vi "GetWhereIsMouseClick.vi"(10 "Coords":T1, 11 "XYGraph输入":refnum<vi>) -> (3 "WhereIsMouse":T2(ring))   [LabVIEW 2015]
uses:
  <vilib>/Utility/miscctls.llb/LVPoint32TypeDef.ctl
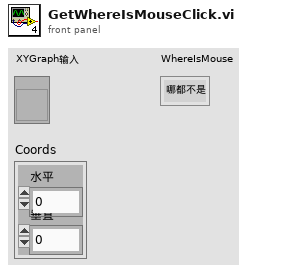
[diagram p1: front panel]
types:
  T1 = typedef "LVPoint32TypeDef.ctl" = cluster{"Horizontal":i32, "Vertical":i32}
  T2 = enum16{"哪都不是", "在曲线上", "在X轴上", "在单Y轴上", "在绘图区域但非曲线上", "在绘图区域上方", "在图例上"}
  T3 = enum16{"哪都不是", "在曲线上", "在X轴上", "在单Y轴上", "在绘图区域但非曲线上"}
  T4 = typedef "LVRectTypeDef.ctl" = cluster{"Left":i16, "Top":i16, "Right":i16, "Bottom":i16}
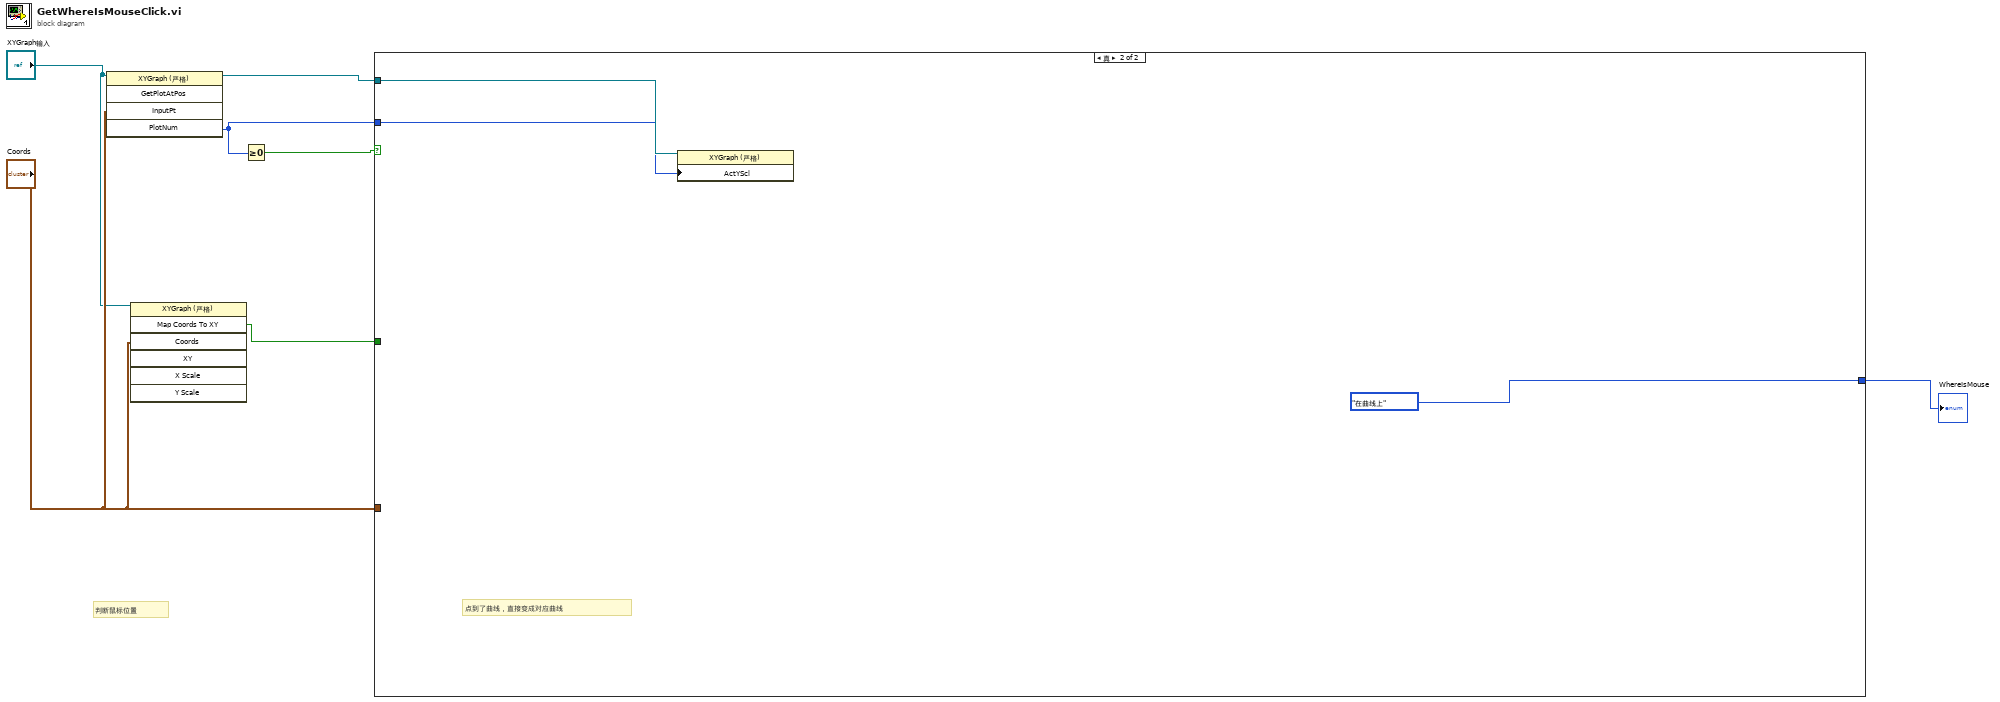
[diagram p0: block diagram]
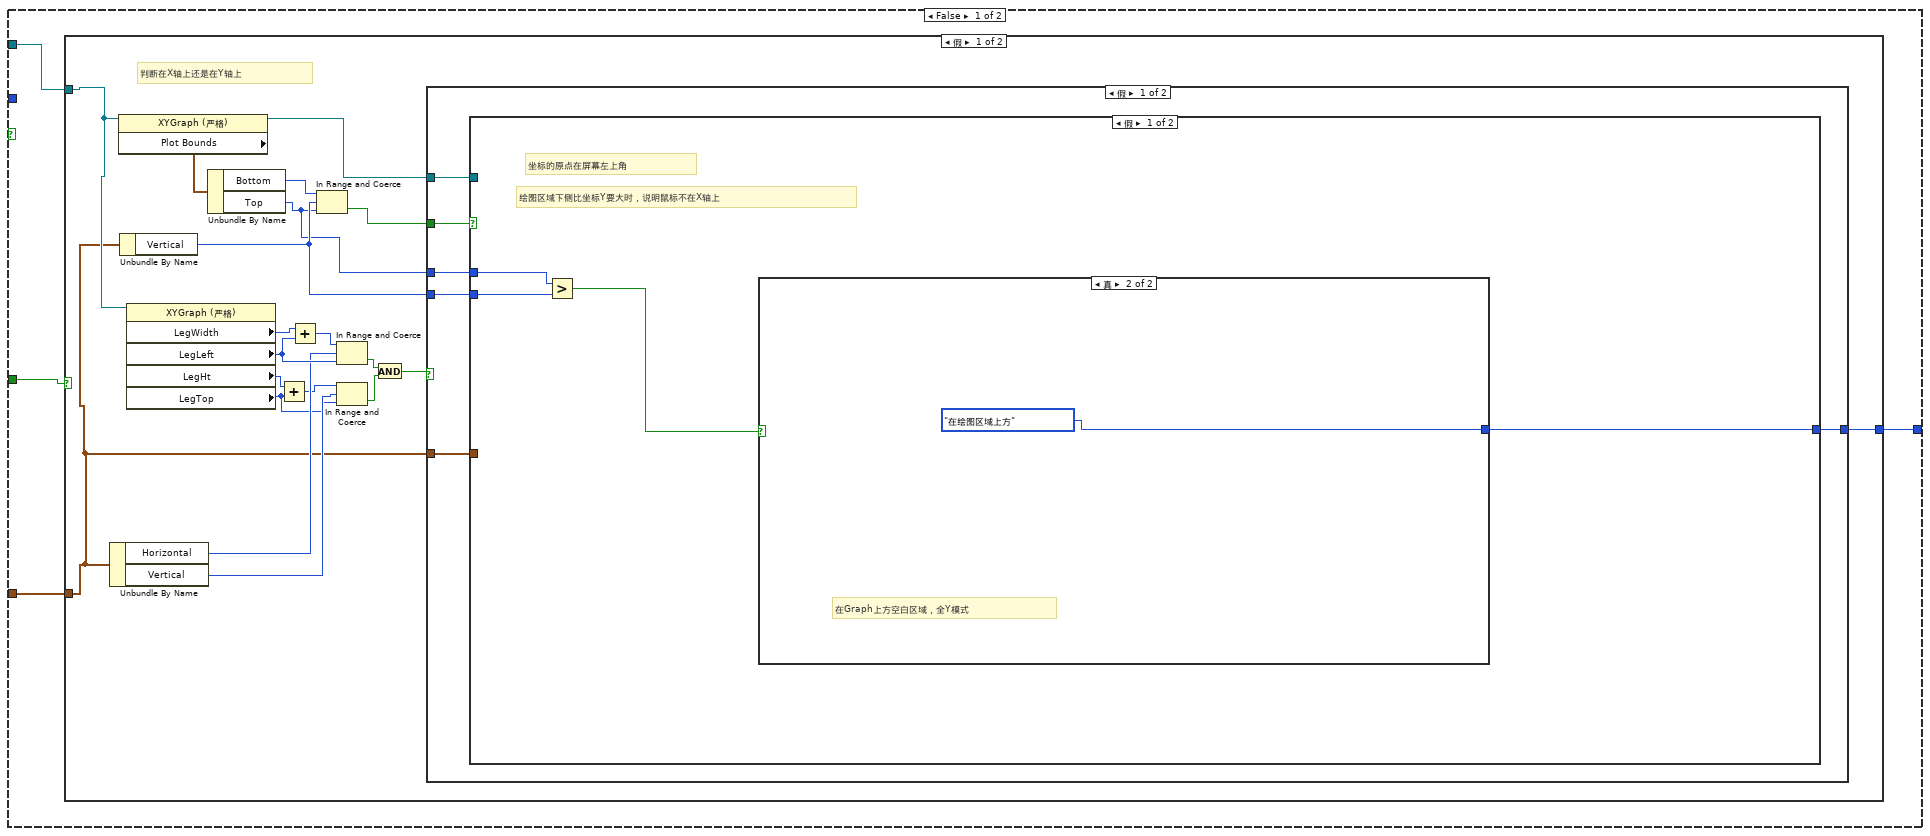
[diagram p2: hidden frame]
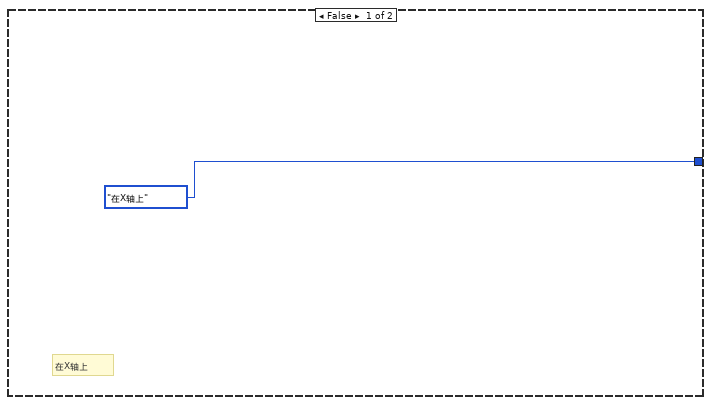
[diagram p3: hidden frame]
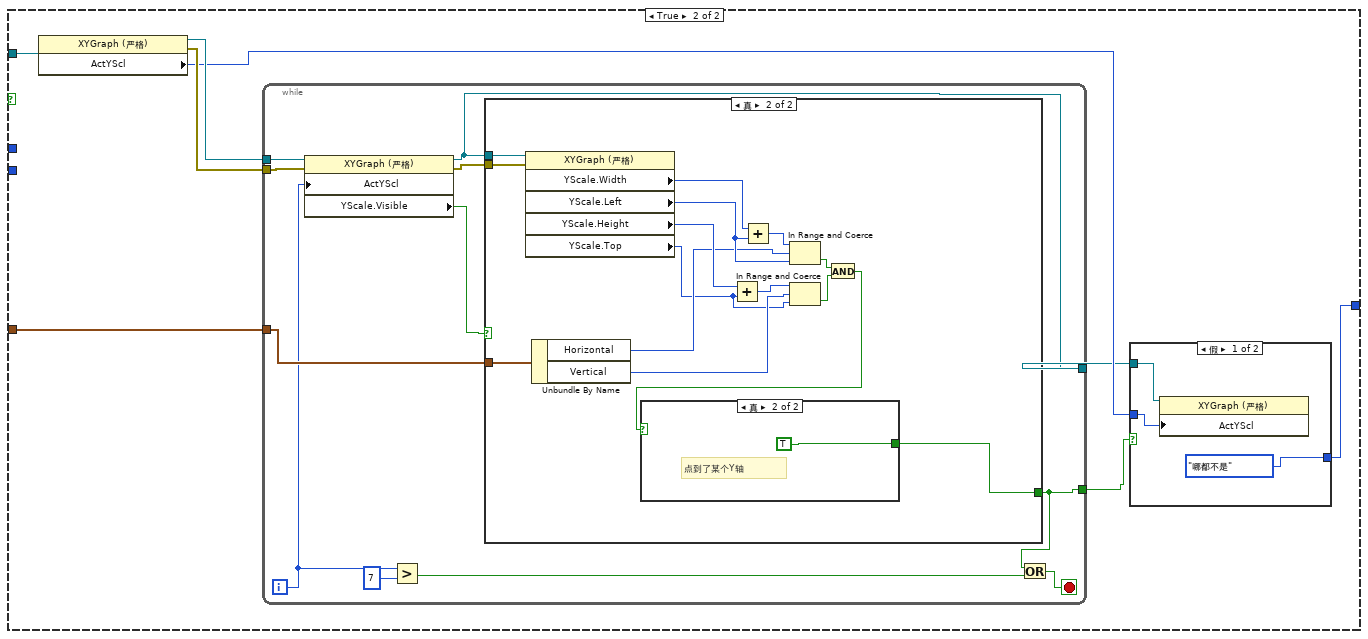
[diagram p4: hidden frame]
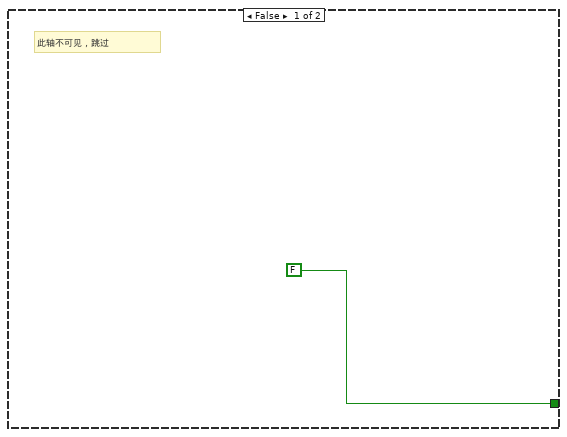
[diagram p5: hidden frame]
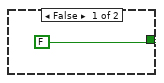
[diagram p6: hidden frame]
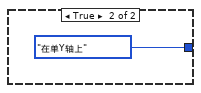
[diagram p7: hidden frame]
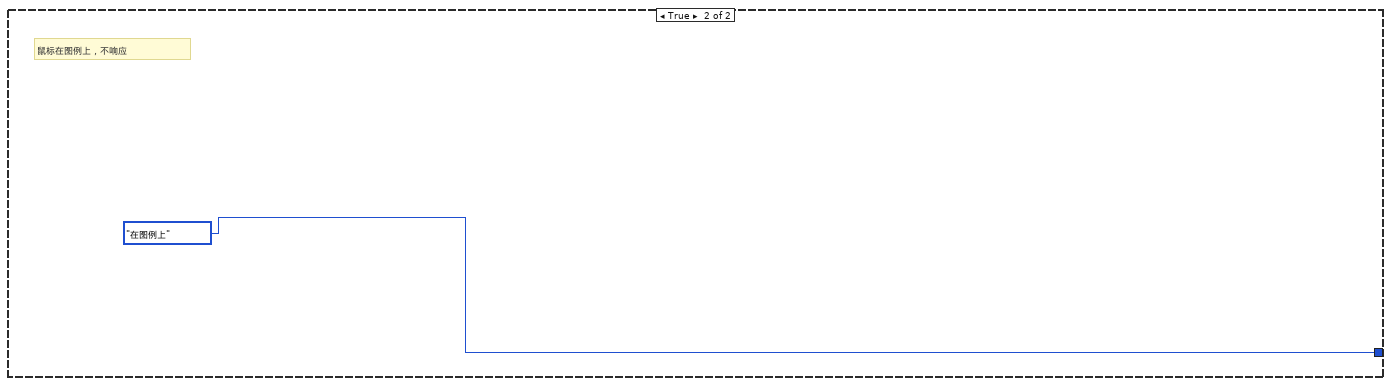
[diagram p8: hidden frame]
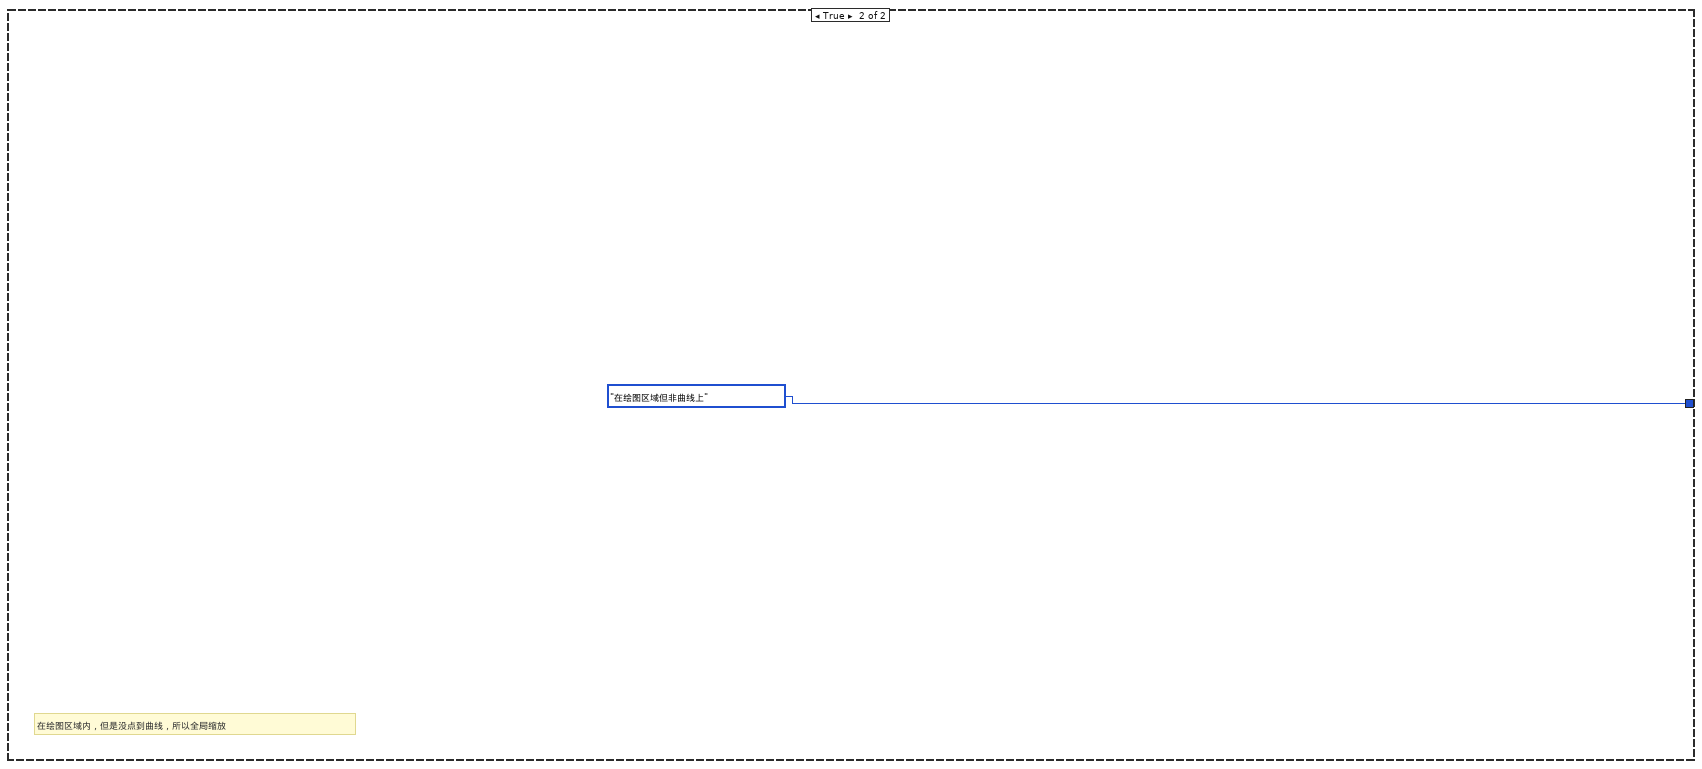
[diagram p9: hidden frame]
diagram:
  # "判断鼠标位置"
  n1 = invoke class="XYGraph (严格)" method="GetPlotAtPos"(reference="XYGraph输入", "InputPt"="Coords") -> (reference out=w2:refnum<vi>, "PlotNum"=w3:i32)  [unwired: 3 in, 3 out]
  n2 = invoke class="XYGraph (严格)" method="Map Coords To XY"(reference="XYGraph输入", "Coords"="Coords") -> ("Map Coords To XY"=w1:bool)  [unwired: 5 in, 6 out]
  n3 = Greater Or Equal To 0?(x=w3) -> (x >= 0?=w4:bool)
  n4 = case shown="真" w4 {
    tunnel: w2 -> [w10 w89]
    tunnel: w3 -> [_ w88]
    tunnel: w1 -> [w11 _]
    tunnel: "Coords" -> [w9 _]
    tunnel: [w8 T2."在曲线上" ("WhereIsMouse")] -> w7
    frame False {
      n5 = case shown="假" w11 {
        tunnel: w10 -> [w31 _]
        tunnel: w9 -> [w20 _]
        tunnel: [w12 T2."在绘图区域但非曲线上" ("WhereIsMouse")] -> w8
        frame False {
          # "判断在X轴上还是在Y轴上"
          n6 = Unbundle By Name(w20) -> ("Horizontal"=w27:i32, "Vertical"=w25:i32)
          n7 = property class="XYGraph (严格)"(reference=w31) -> (reference out=w21:refnum<vi>, "Plot Bounds"=w19:T4)  [unwired: 1 in, 1 out]
          n8 = Unbundle By Name(w20) -> ("Vertical"=w14:i32)
          n9 = property class="XYGraph (严格)"(reference=w31) -> ("LegWidth"=w30:u32, "LegLeft"=w28:i32, "LegHt"=w26:u32, "LegTop"=w18:i32)  [unwired: 1 in, 2 out]
          n10 = Unbundle By Name(w19) -> ("Bottom"=w16:i16, "Top"=w13:i16)
          n11 = Add(x=w26, y=w18) -> (x+y=w17:u32)
          n12 = Add(x=w30, y=w28) -> (x+y=w29:u32)
          n13 = In Range and Coerce(upper limit=w16, x=w14, lower limit=w13) -> (In Range?=w15:bool)  [unwired: 1 out]
          n14 = In Range and Coerce(upper limit=w29, x=w27, lower limit=w28) -> (In Range?=w24:bool)  [unwired: 1 out]
          n15 = In Range and Coerce(upper limit=w17, x=w25, lower limit=w18) -> (In Range?=w23:bool)  [unwired: 1 out]
          n16 = And(x=w24, y=w23) -> (x .and. y?=w22:bool)
          n17 = case shown="假" w22 {
            tunnel: w15 -> [w37 _]
            tunnel: w21 -> [w36 _]
            tunnel: w20 -> [w35 _]
            tunnel: w14 -> [w34 _]
            tunnel: w13 -> [w33 _]
            tunnel: [w32 T2."在图例上" ("WhereIsMouse")] -> w12
            frame False {
              n18 = case shown="假" w37 {
                tunnel: w36 -> [_ w51]
                tunnel: w35 -> [_ w48]
                tunnel: w34 -> [w39 _]
                tunnel: w33 -> [w40 _]
                tunnel: [w38 w45] -> w32
                frame False {
                  # "绘图区域下侧比坐标Y要大时，说明鼠标不在X轴上"
                  # "坐标的原点在屏幕左上角"
                  n19 = Greater?(x=w40, y=w39) -> (0:w41:bool)
                  n20 = case shown="真" w41 {
                    tunnel: [T2."在X轴上" ("WhereIsMouse") T2."在绘图区域上方" ("WhereIsMouse")] -> w38
                    frame False {
                      # "在X轴上"
                    }
                    frame True {
                      # "在Graph上方空白区域，全Y模式"
                    }
                  }
                }
                frame True {
                  n21 = property class="XYGraph (严格)"(reference=w51) -> (reference out=w50:refnum<vi>, error out=w49:errorcluster, "ActYScl"=w47:i32)  [unwired: 1 in]
                  n22 = while {
                    tunnel: w50 -> [w62]
                    tunnel: w49 -> [w60]
                    tunnel: w48 -> [w58]
                    tunnel: [w57] -> w46
                    tunnel: [w52] -> w44
                    i -> [w56]
                    stop <- w54 stop-if-true
                    n23 = property class="XYGraph (严格)"(reference=w62, error in=w60, "ActYScl"=w56) -> (reference out=w57:refnum<vi>, error out=w61:errorcluster, "YScale.Visible"=w59:bool)
                    n24 = Greater?(x=w56, y=7) -> (0:w53:bool)
                    n25 = case shown="真" w59 {
                      tunnel: w57 -> [_ w73]
                      tunnel: w61 -> [_ w72]
                      tunnel: w58 -> [_ w70]
                      tunnel: [FALSE w64] -> w52
                      frame False {
                        # "此轴不可见，跳过"
                      }
                      frame True {
                        n26 = property class="XYGraph (严格)"(reference=w73, error in=w72) -> ("YScale.Width"=w75:u32, "YScale.Left"=w74:i32, "YScale.Height"=w71:u32, "YScale.Top"=w65:i32)  [unwired: 2 out]
                        n27 = Unbundle By Name(w70) -> ("Horizontal"=w69:i32, "Vertical"=w68:i32)
                        n28 = Add(x=w71, y=w65) -> (x+y=w66:u32)
                        n29 = Add(x=w75, y=w74) -> (x+y=w76:u32)
                        n30 = In Range and Coerce(upper limit=w76, x=w69, lower limit=w74) -> (In Range?=w77:bool)  [unwired: 1 out]
                        n31 = In Range and Coerce(upper limit=w66, x=w68, lower limit=w65) -> (In Range?=w78:bool)  [unwired: 1 out]
                        n32 = And(x=w77, y=w78) -> (x .and. y?=w67:bool)
                        n33 = case shown="真" w67 {
                          tunnel: [FALSE TRUE] -> w64
                          frame False {
                          }
                          frame True {
                            # "点到了某个Y轴"
                          }
                        }
                      }
                    }
                    n34 = Or(x=w52, y=w53) -> (x .or. y?=w54:bool)
                  }
                  n35 = case shown="假" w44 {
                    tunnel: w47 -> [w82 _]
                    tunnel: w46 -> [w83 _]
                    tunnel: [T2."哪都不是" ("WhereIsMouse") T3."在单Y轴上" ("WhereIsMouse")] -> w45
                    frame False {
                      n36 = property class="XYGraph (严格)"(reference=w83, "ActYScl"=w82) -> ()  [unwired: 1 in, 2 out]
                    }
                    frame True {
                    }
                  }
                }
              }
            }
            frame True {
              # "鼠标在图例上，不响应"
            }
          }
        }
        frame True {
          # "在绘图区域内，但是没点到曲线，所以全局缩放"
        }
      }
    }
    frame True {
      # "点到了曲线，直接变成对应曲线"
      n37 = property class="XYGraph (严格)"(reference=w89, "ActYScl"=w88) -> ()  [unwired: 1 in, 2 out]
    }
  }
  "WhereIsMouse" <- w7
